vi "Drive_Loop_Command.vi"   [LabVIEW 2016]
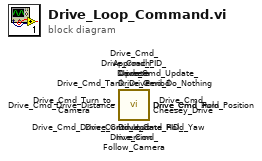
[diagram p0: block diagram]
diagram:
  n1 = call <userlib>:"Drive_Cmd_Update_PID_Inversion.vi"() -> ()  [unwired: 12 in]
  n2 = call <userlib>:"Drive_Cmd_Update_Period.vi"() -> ()  [unwired: 12 in]
  n3 = call <userlib>:"Drive_Cmd_Turn_to_Camera.vi"() -> ()  [unwired: 11 in, 1 out]
  n4 = call <userlib>:"Drive_Cmd_Turn.vi"() -> ()  [unwired: 11 in, 1 out]
  n5 = call <userlib>:"Drive_Cmd_Tank_Drive.vi"() -> ()  [unwired: 11 in, 1 out]
  n6 = call <userlib>:"Drive_Cmd_PID_Update.vi"() -> ()  [unwired: 12 in]
  n7 = call <userlib>:"Drive_Cmd_Hold_Yaw.vi"() -> ()  [unwired: 11 in, 1 out]
  n8 = call <userlib>:"Drive_Cmd_Hold_Position.vi"() -> ()  [unwired: 11 in, 1 out]
  n9 = call <userlib>:"Drive_Cmd_Follow_Camera.vi"() -> ()  [unwired: 11 in, 1 out]
  n10 = call <userlib>:"Drive_Cmd_Drive_Distance.vi"() -> ()  [unwired: 11 in, 1 out]
  n11 = call <userlib>:"Drive_Cmd_Drive_Continuous.vi"() -> ()  [unwired: 11 in, 1 out]
  n12 = call <userlib>:"Drive_Cmd_Do_Nothing.vi"() -> ()  [unwired: 12 in]
  n13 = call <userlib>:"Drive_Cmd_Cheesey_Drive.vi"() -> ()  [unwired: 11 in, 1 out]
  n14 = call <userlib>:"Drive_Cmd_Approach_Camera.vi"() -> ()  [unwired: 11 in, 1 out]
